vi "Write remote port.vi"(8 "error in (no error)":errorcluster, 10 "remote port (80)":u16=80, 11 "TCPConnection in":refnum<class "TCPConnection.lvclass">) -> (0 "error out":errorcluster, 3 "TCPConnection out":refnum<class "TCPConnection.lvclass">)   [LabVIEW 2013, in "MQTT_TCP.lvlib" / "TCPConnection.lvclass"]
uses:
  TCPConnection.lvclass
  TCPConnection.lvclass/TCPConnection.ctl
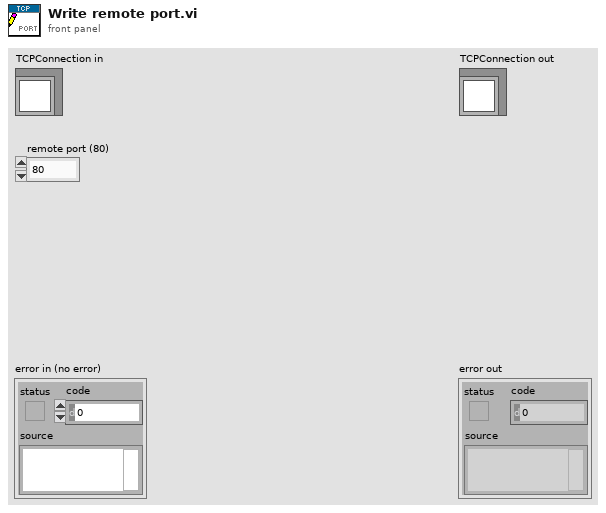
[diagram p1: front panel]
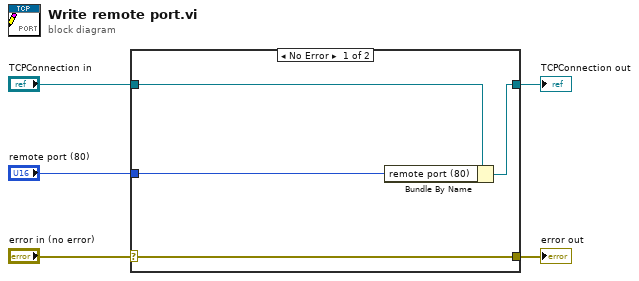
[diagram p0: block diagram]
diagram:
  n1 = case shown="No Error" "error in (no error)" {
    selector: "error in (no error)" -> [w9 w10]
    tunnel: [w9 w10] -> w4
    tunnel: [w7 w11] -> w2
    tunnel: "TCPConnection in" -> [w8 w11]
    tunnel: "remote port (80)" -> [w6 _]
    frame No Error {
      n2 = Bundle By Name(cluster=w8, "remote port (80)"=w6) -> (w7:refnum<class "TCPConnection.lvclass">)
    }
    frame Error {
    }
  }
  "error out" <- w4
  "TCPConnection out" <- w2
